vi "PS90_PosMode.vi"(5 "read?":bool, 7 "Control unit ID":i32=1 min=1 max=10, 8 "error in (no error)":errorcluster, 9 "Value-In":i32 min=0 max=1, 10 "Axis number":i32=1 min=1 max=9, 11 "DLOwis.lvclass":refnum<class "DLOwis.lvclass">) -> (0 "error out":errorcluster, 1 "Value-Out":i32, 3 "DLOwis.lvclass":refnum<class "DLOwis.lvclass">)   [LabVIEW 2018, in "DLOwis.lvclass"]
doc: "PS90_PosMode.vi, created: 17.10.2006 alex; last change: 19.07.2016 alex;\n\n<B>FUNCTIONS:</B> \n\n<B>Read:</B> FALSE: read positioning mode of an axis.\n<B>Write:</B> TRUE: set positioning mode of an axis.\n----------------------------------------------------------------------------------------\n<B>INPUT:</B>\n[TF] <B>function:</B> function selector. (Read, Write)\n[I32] <B>Control unit ID:</B> control unit index. (Default=1, Range=1...10)\n[I32] <B>Axis number:</B> axis number. (Default=1, Range=1...9)\n[I32] <B>Value-In:</B> positioning mode. (only for Write: Default=0, Range=0...1)\n0 - trapezoidal profile,\n1 - S-curve profile. \n[CLU] <B>error in</B>\n----------------------------------------------------------------------------------------\n<B>OUTPUT:</B>\n[I32] <B>Value-Out:</B> positioning mode. (for Write: Value-Out=Value-In)\n0 - trapezoidal profile is active,\n1 - S-curve profile is active.\n[CLU] <B>error out</B>\n----------------------------------------------------------------------------------------\n<B>SUB-VIs:</B>\nPS90_GetReadError.vi\n----------------------------------------------------------------------------------------\n<B>EXT-Calls:</B>\nps90.dll (V2.00)\n----------------------------------------------------------------------------------------"
uses:
  DLOwis.lvclass
  C:/Users/Sergey Denisov/Documents/REPS/TRANCON/Classes/Delay Line/DelayLine.lvclass
  DelayLine.lvclass/DelayLine.ctl
  DelayLine.lvclass
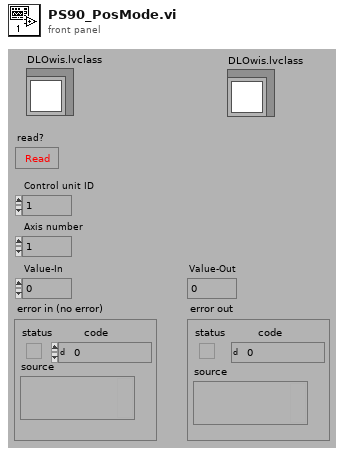
[diagram p1: front panel]
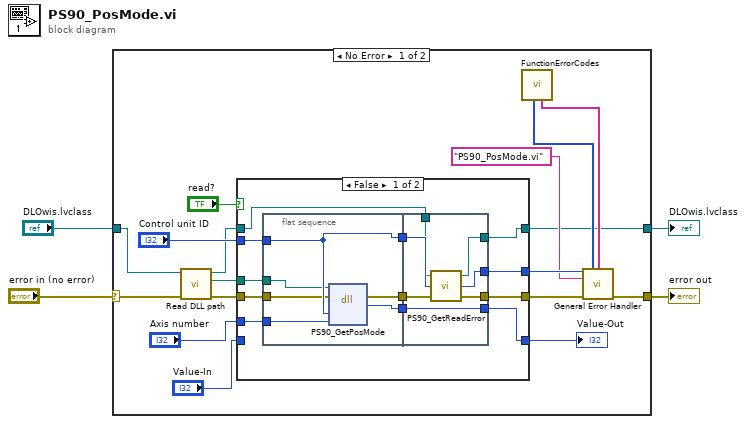
[diagram p0: block diagram]
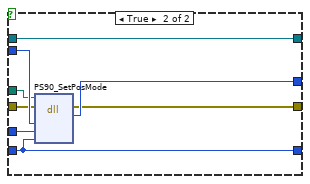
[diagram p2: hidden frame]
diagram:
  n1 = case shown="No Error" "error in (no error)" {
    selector: "error in (no error)" -> [w7 w55]
    tunnel: [w21 w55] -> w4
    tunnel: [w5 w56] -> w2
    tunnel: "DLOwis.lvclass" -> [w8 w56]
    frame No Error {
      n2 = call "Read DLL path.vi"("error in (no error)"=w7, "DelayLine in"=w8) -> ("error out"=w10:errorcluster, "DLL path"=w9:path, "DelayLine out"=w6:refnum<class "DLOwis.lvclass">)  [unwired: 7 in]
      n3 = case shown="False" "read?" {
        tunnel: "Control unit ID" -> [w32 w53]
        tunnel: [w33 w54] -> w18
        tunnel: "Value-In" -> [_ w51]
        tunnel: [w31 w51] -> w16
        tunnel: "Axis number" -> [w30 w52]
        tunnel: [w25 w50] -> w11
        tunnel: w10 -> [w27 w49]
        tunnel: w9 -> [w22 w48]
        tunnel: w6 -> [w24 w47]
        tunnel: [w23 w47] -> w5
        frame False {
          n4 = flat-sequence {
            tunnel: w32 -> [w39]
            tunnel: [w39] -> w29
            tunnel: [w38] -> w28
            tunnel: w30 -> [w37]
            tunnel: w27 -> [w36]
            tunnel: [w35] -> w26
            tunnel: w22 -> [w34]
            tunnel: [w46] -> w33
            tunnel: w29 -> [w45]
            tunnel: [w44] -> w31
            tunnel: w28 -> [w44]
            tunnel: w26 -> [w43]
            tunnel: [w42] -> w25
            tunnel: w24 -> [w41]
            tunnel: [w40] -> w23
            frame #0 {
              n5 = dll-call lib="C:/Users/Sergey Denisov/Documents/REPS/TRANCON/DLL/ps90.dll" fn="PS90_GetPosMode" label="PS90_\nGetPos\nMode"(path in=w34, error in=w36, "Index"=w39, "AxisNr"=w37) -> (error out=w35:errorcluster, "Rückgabetyp"=w38:i32)  [unwired: 3 in, 1 out]
            }
            frame #1 {
              n6 = call "PS90_GetReadError.vi"("error in (no error)"=w43, "Control unit ID"=w45, "DLOwis.lvclass"=w41) -> ("error IO"=w42:errorcluster, "Read error"=w46:i32, "DLOwis.lvclass"=w40:refnum<class "DLOwis.lvclass">)
            }
          }
        }
        frame True {
          n7 = dll-call lib="C:/Users/Sergey Denisov/Documents/REPS/TRANCON/DLL/ps90.dll" fn="PS90_SetPosMode" label="PS90_\nSetPos\nMode"(path in=w48, error in=w49, "Index"=w53, "AxisNr"=w52, "Value"=w51) -> (error out=w50:errorcluster, "Rückgabetyp"=w54:i32)  [unwired: 4 in, 1 out]
        }
      }
      "Value-Out" <- w16
      n8 = call "FunctionErrorCodes.vi"() -> ("[user-defined codes]"=w13:i32[], "[user-defined descriptions]"=w12:string[])  [unwired: 8 in]
      n9 = call <vilib>:"General Error Handler.vi"("[error code] (0)"=w18, "[user-defined codes]"=w13, "[user-defined descriptions]"=w12, "[error source] (\" \")"="PS90_PosMode.vi" ("[error source] (\" \")"), "error in (no error)"=w11) -> ("error out"=w21:errorcluster)  [unwired: 6 in, 4 out]
    }
    frame Error {
    }
  }
  "error out" <- w4
  "DLOwis.lvclass" <- w2
